vi "Start + Stop Sift Proxy.vi"() -> (0 "Error":errorcluster, 2 "Success":bool)   [LabVIEW 2024]
uses:
  Sift API/Sift Client.lvclass
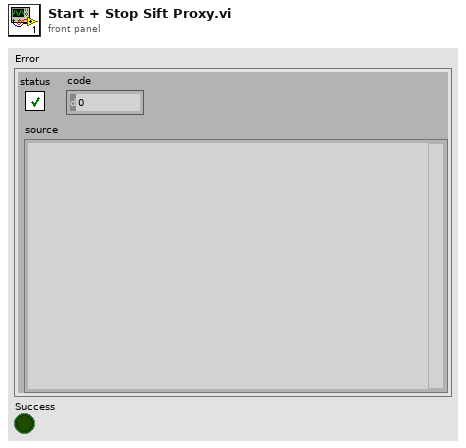
[diagram p1: front panel]
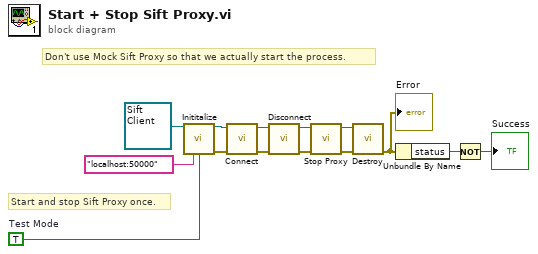
[diagram p0: block diagram]
diagram:
  w13 = TRUE  # Test Mode
  # "Don't use Mock Sift Proxy so that we actually start the process."
  # "Start and stop Sift Proxy once."
  n1 = call-dynamic "Inititalize.vi"("Sift Client in"=refnum<class "Sift Client.lvclass"> refnum ("Sift Client.lvlib:Sift Client.lvclass"), "Sift Proxy Address"="localhost:50000", "Test Mode"=w13) -> ("Sift Client out"=w10:refnum<class "Sift Client.lvclass">, "error out"=w9:errorcluster)  [unwired: 11 in]
  n2 = call-dynamic "Connect.vi"("error in (no error)"=w9, "Sift Client in"=w10) -> ("error out"=w11:errorcluster, "Sift Client out"=w12:refnum<class "Sift Client.lvclass">)  [unwired: 7 in, 1 out]
  n3 = call-dynamic "Disconnect.vi"("error in (no error)"=w11, "Sift Client in"=w12) -> ("error out"=w6:errorcluster, "Sift Client out"=w8:refnum<class "Sift Client.lvclass">)  [unwired: 8 in]
  n4 = call-dynamic "Stop Proxy.vi"("error in (no error)"=w6, "Sift Client in"=w8) -> ("error out"=w5:errorcluster, "Sift Client out"=w7:refnum<class "Sift Client.lvclass">)  [unwired: 8 in]
  n5 = call-dynamic "Destroy.vi"("error in (no error)"=w5, "Sift Client in"=w7) -> ("error out"=w4:errorcluster)  [unwired: 8 in, 1 out]
  "Error" <- w4
  n6 = Unbundle By Name(w4) -> ("status"=w3:bool)
  n7 = Not(x=w3) -> (.not. x?=→"Success":bool)
